vi "mediaIntesecaoCameras_v2.vi"(11 "Cameras Array":T1[](array[typedef]) {"robots_blue"."height" format="%+4.3f"; "robots_blue"."pixel_y" format="%+4.3f"; "robots_blue"."pixel_x" format="%+4.3f"; "robots_blue"."orientation" format="%+4.3f"; "robots_blue"."y" format="%+4.3f"; "robots_blue"."confidence" format="%4.3f"; "robots_blue"."x" format="%+4.3f"; "robots_yellow"."height" format="%+4.3f"; "robots_yellow"."pixel_y" format="%+4.3f"; "robots_yellow"."pixel_x" format="%+4.3f"; "robots_yellow"."orientation" format="%+4.3f"; "robots_yellow"."y" format="%+4.3f"; "robots_yellow"."confidence" format="%4.3f"; "robots_yellow"."x" format="%+4.3f"}) -> (3 "frame out":T1 {"robots_blue"."height" format="%+4.3f"; "robots_blue"."pixel_y" format="%+4.3f"; "robots_blue"."pixel_x" format="%+4.3f"; "robots_blue"."orientation" format="%+4.3f"; "robots_blue"."y" format="%+4.3f"; "robots_blue"."confidence" format="%4.3f"; "robots_blue"."x" format="%+4.3f"; "robots_yellow"."height" format="%+4.3f"; "robots_yellow"."pixel_y" format="%+4.3f"; "robots_yellow"."pixel_x" format="%+4.3f"; "robots_yellow"."orientation" format="%+4.3f"; "robots_yellow"."y" format="%+4.3f"; "robots_yellow"."confidence" format="%4.3f"; "robots_yellow"."x" format="%+4.3f"})   [LabVIEW 2018]
uses:
  SSL Detection Frame.ctl
  SSL Detection Robot.ctl
  <vilib>/Analysis/Matrix/Datatypes/RealMatrix.ctl
  SSL Detection Ball.ctl
  <vilib>/Analysis/Matrix/NI_Matrix.lvlib
panel:
  in  "Unico frame":T1 {"robots_blue"."height" format="%+4.3f"; "robots_blue"."pixel_y" format="%+4.3f"; "robots_blue"."pixel_x" format="%+4.3f"; "robots_blue"."orientation" format="%+4.3f"; "robots_blue"."y" format="%+4.3f"; "robots_blue"."confidence" format="%4.3f"; "robots_blue"."x" format="%+4.3f"; "robots_yellow"."height" format="%+4.3f"; "robots_yellow"."pixel_y" format="%+4.3f"; "robots_yellow"."pixel_x" format="%+4.3f"; "robots_yellow"."orientation" format="%+4.3f"; "robots_yellow"."y" format="%+4.3f"; "robots_yellow"."confidence" format="%4.3f"; "robots_yellow"."x" format="%+4.3f"}
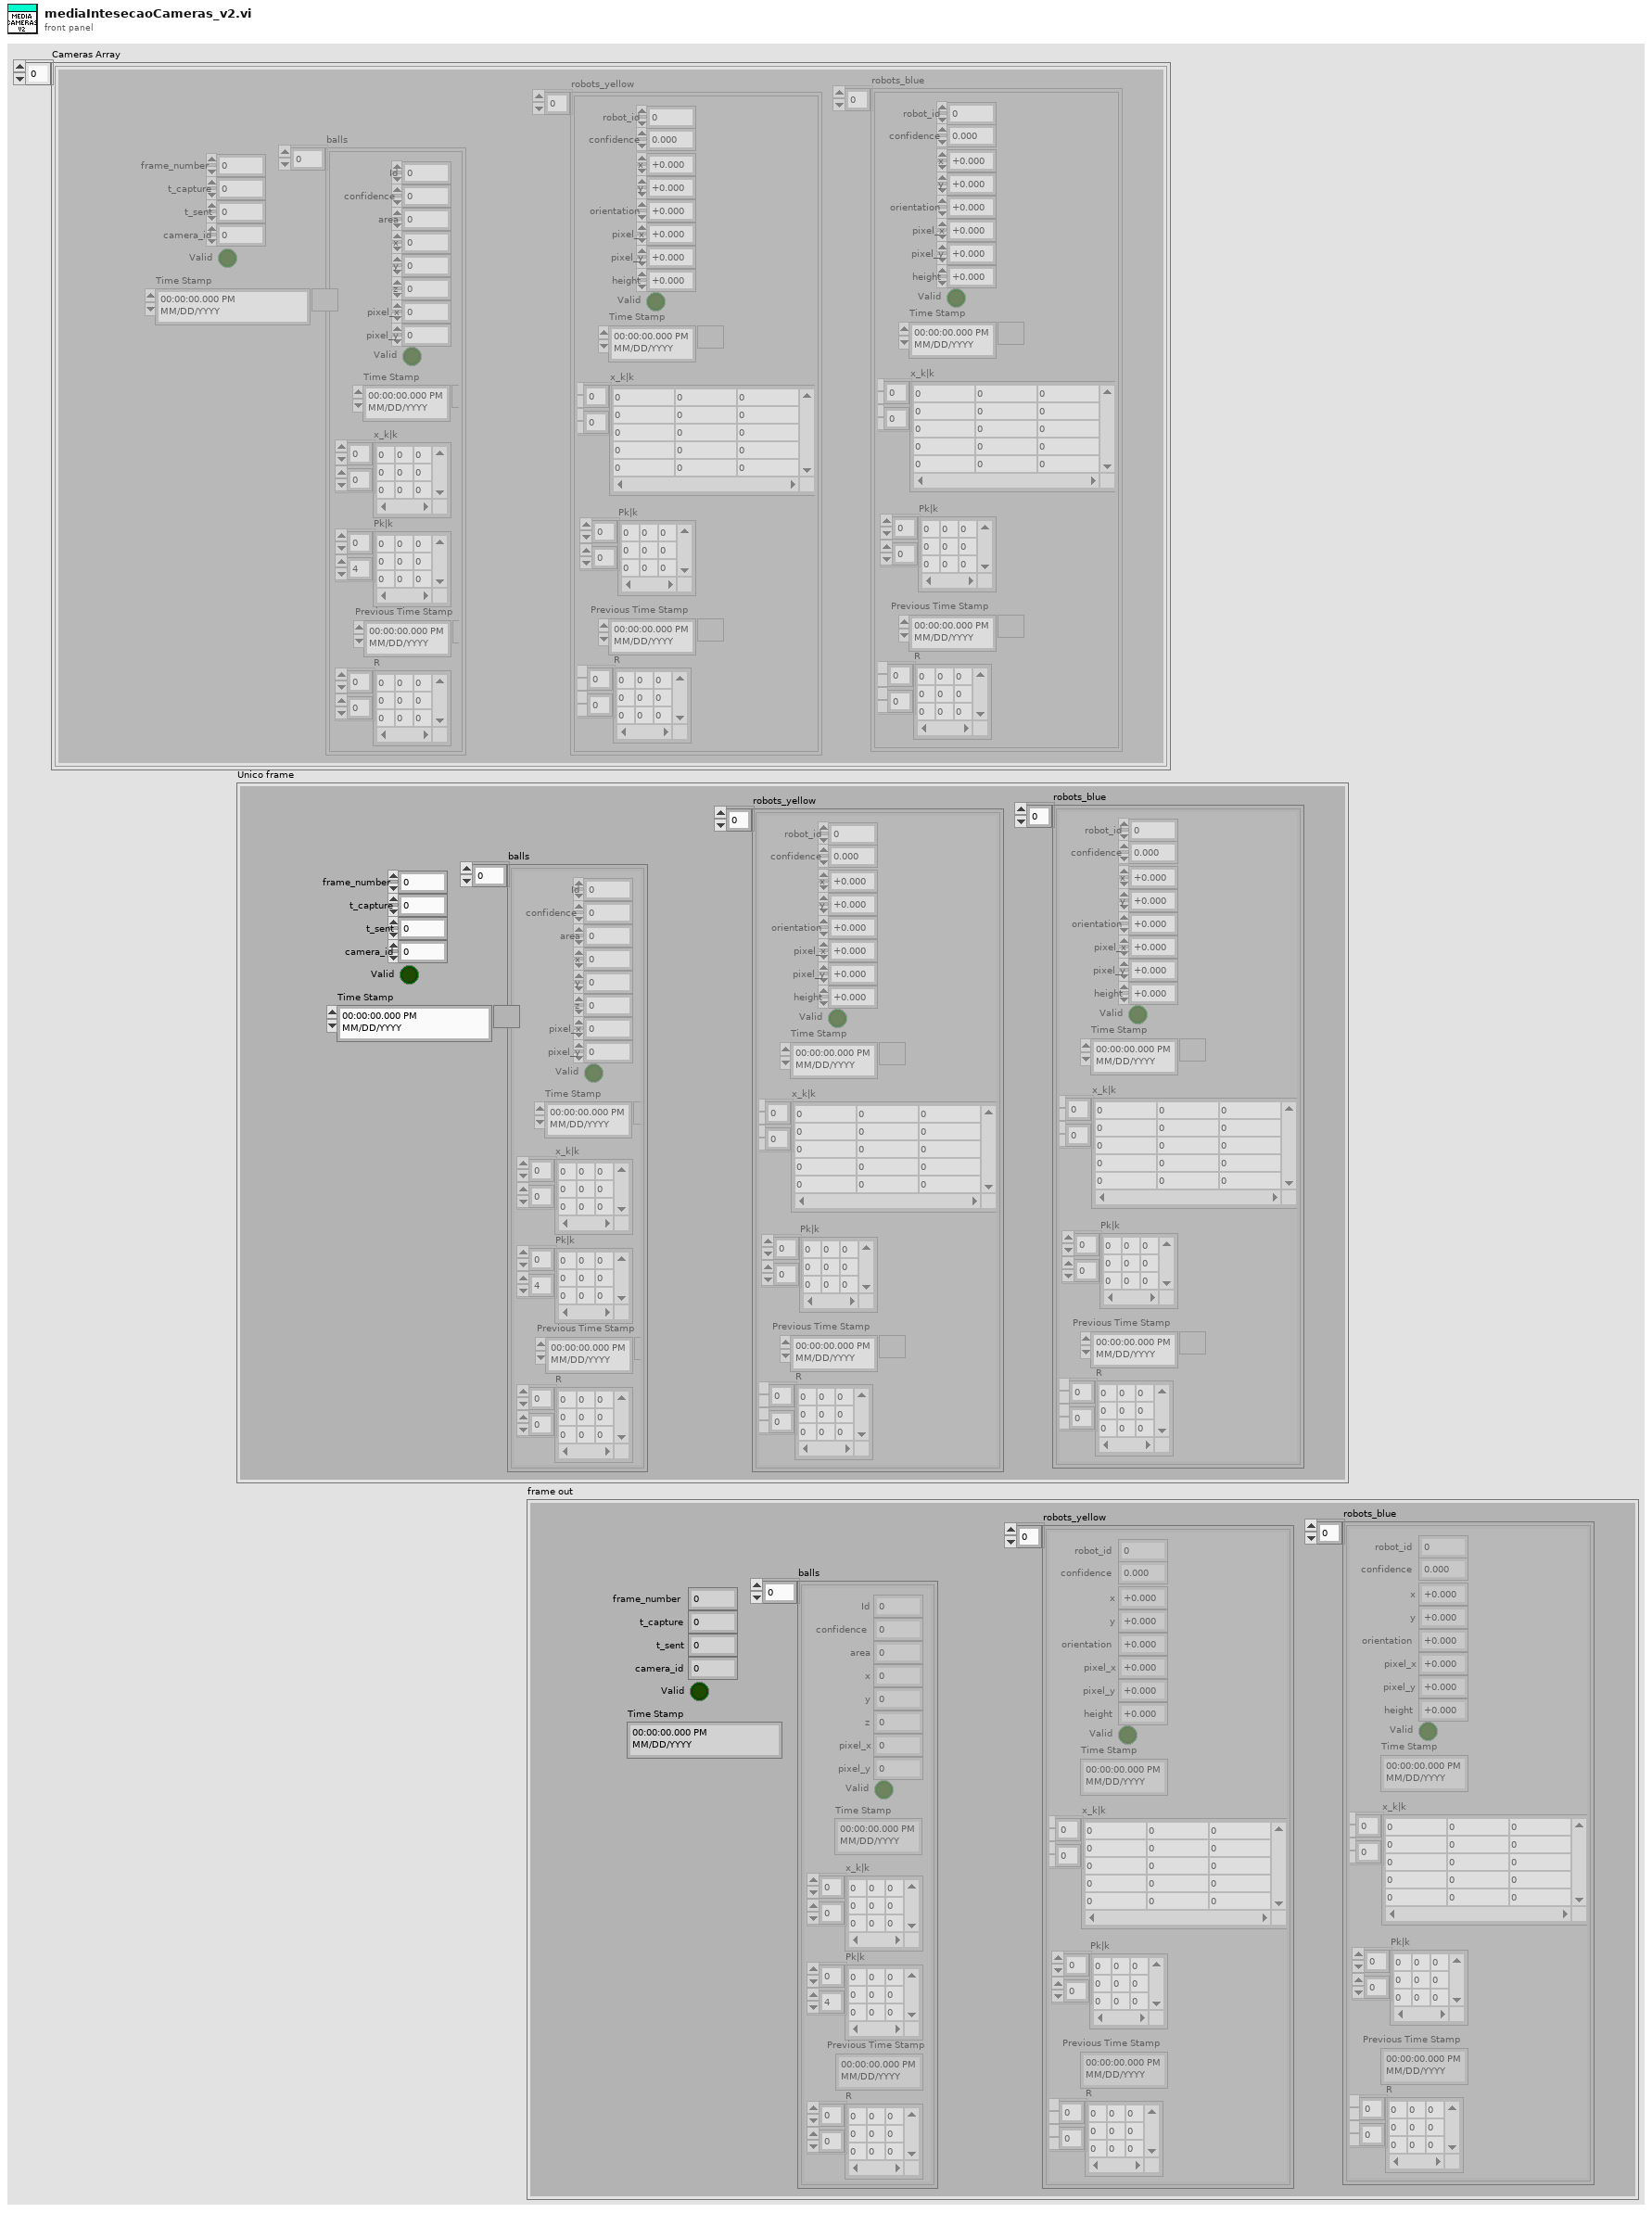
[diagram p1: front panel]
types:
  T1 = typedef "SSL Detection Frame.ctl" = cluster{"frame_number":u32, "t_capture":dbl, "t_sent":dbl, "camera_id":u32, "robots_yellow":T2[], "robots_blue":T2[], "balls":T4[], "Valid":bool, "Time Stamp":timestamp}
  T2 = typedef "SSL Detection Robot.ctl" = cluster{"x":sgl, "robot_id":u32, "confidence":sgl, "y":sgl, "orientation":sgl, "pixel_x":sgl, "pixel_y":sgl, "height":sgl, "Valid":bool, "Time Stamp":timestamp, "x_k|k":T3, "Pk|k":T3, "Previous Time Stamp":timestamp, "R":T3}
  T3 = typedef "NI_Matrix.lvlib/RealMatrix.ctl" = dbl[][]
  T4 = typedef "SSL Detection Ball.ctl" = cluster{"x":sgl, "area":u32, "confidence":sgl, "y":sgl, "z":sgl, "pixel_x":sgl, "pixel_y":sgl, "Valid":bool, "Time Stamp":timestamp, "x_k|k":T3, "Pk|k":T3, "Id":u32, "Previous Time Stamp":timestamp, "R":T3}
  T5 = cluster{"x":sgl, "y":sgl, "orientation":sgl, "robot_id":u32, "camera_id":u32}
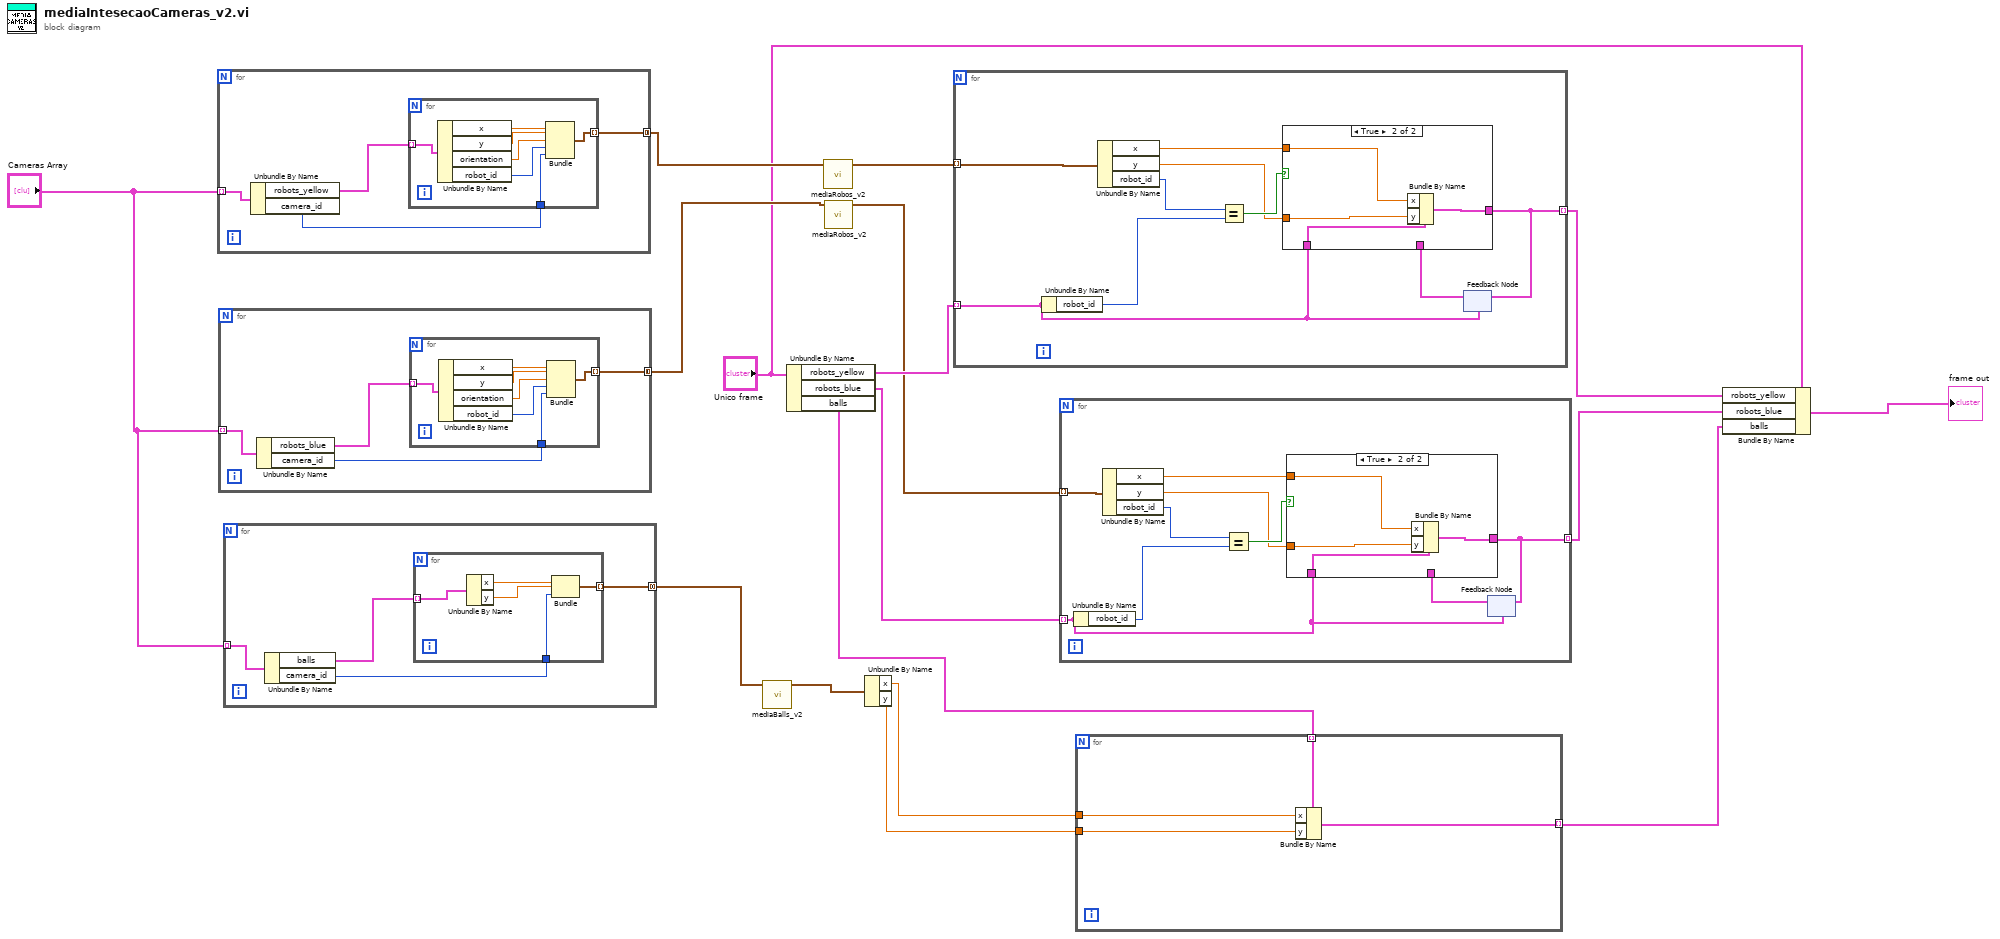
[diagram p0: block diagram]
diagram:
  n1 = for {
    tunnel: "Cameras Array" -> [w21] mode=indexing
    tunnel: [w19] -> w17 mode=concatenating
    n2 = Unbundle By Name(w21) -> ("robots_yellow"=w20:T2[], "camera_id"=w18:u32)
    n3 = for {
      tunnel: w20 -> [w28] mode=indexing
      tunnel: [w25] -> w19 mode=indexing
      tunnel: w18 -> [w22]
      n4 = Unbundle By Name(w28) -> ("x"=w27:sgl, "y"=w26:sgl, "orientation"=w24:sgl, "robot_id"=w23:u32)
      n5 = Bundle("x"=w27, "y"=w26, "orientation"=w24, "robot_id"=w23, "camera_id"=w22) -> (w25:T5)  [unwired: 1 in]
    }
  }
  n6 = for {
    tunnel: "Cameras Array" -> [w32] mode=indexing
    tunnel: [w31] -> w12 mode=concatenating
    n7 = Unbundle By Name(w32) -> ("robots_blue"=w29:T2[], "camera_id"=w30:u32)
    n8 = for {
      tunnel: w29 -> [w39] mode=indexing
      tunnel: [w36] -> w31 mode=indexing
      tunnel: w30 -> [w33]
      n9 = Unbundle By Name(w39) -> ("x"=w38:sgl, "y"=w37:sgl, "orientation"=w35:sgl, "robot_id"=w34:u32)
      n10 = Bundle("x"=w38, "y"=w37, "orientation"=w35, "robot_id"=w34, "camera_id"=w33) -> (w36:T5)  [unwired: 1 in]
    }
  }
  n11 = for {
    tunnel: "Cameras Array" -> [w43] mode=indexing
    tunnel: [w42] -> w6 mode=concatenating
    n12 = Unbundle By Name(w43) -> ("balls"=w40:T4[], "camera_id"=w41:u32)
    n13 = for {
      tunnel: w40 -> [w48] mode=indexing
      tunnel: [w45] -> w42 mode=indexing
      tunnel: w41 -> [w44]
      n14 = Unbundle By Name(w48) -> ("x"=w47:sgl, "y"=w46:sgl)
      n15 = Bundle("x"=w47, "y"=w46, "camera_id"=w44) -> (w45:cluster{"x":sgl, "y":sgl, "camera_id":u32})  [unwired: 1 in]
    }
  }
  n16 = call "mediaBalls_v2.vi"("Array Ball Pose + CamID"=w6) -> ("Ball out"=w5:cluster{"x":dbl, "y":dbl})  [unwired: 10 in]
  n17 = Unbundle By Name("Unico frame") -> ("robots_yellow"=w16:T2[], "robots_blue"=w14:T2[], "balls"=w4:T4[])
  n18 = call "mediaRobos_v2.vi"("Array Robot Pose + CamID"=w17) -> ("Array"=w15:cluster{"x":dbl, "y":dbl, "robot_id":i32}[])  [unwired: 10 in]
  n19 = call "mediaRobos_v2.vi"("Array Robot Pose + CamID"=w12) -> ("Array"=w13:cluster{"x":dbl, "y":dbl, "robot_id":i32}[])  [unwired: 10 in]
  n20 = Unbundle By Name(w5) -> ("x"=w3:dbl, "y"=w2:dbl)
  n21 = for {
    tunnel: w16 -> [w49] mode=indexing
    tunnel: w15 -> [w56] mode=indexing
    tunnel: [w51] -> w10 mode=indexing
    n22 = Unbundle By Name(w49) -> ("robot_id"=w57:u32)
    n23 = Unbundle By Name(w56) -> ("x"=w53:dbl, "y"=w52:dbl, "robot_id"=w55:i32)
    n24 = Equal?(x=w55, y=w57) -> (x = y?=w54:bool)
    n25 = feedback #1(w49) -> (w50:T2)
    n26 = case shown="True" w54 {
      tunnel: w49 -> [_ w62]
      tunnel: w53 -> [_ w61]
      tunnel: w52 -> [_ w60]
      tunnel: [w58 w59] -> w51
      tunnel: w50 -> [w58 _]
      frame False {
      }
      frame True {
        n27 = Bundle By Name(cluster=w62, "x"=w61, "y"=w60) -> (w59:T2)
      }
    }
    n28 = feedback-in #1(w51) -> ()
  }
  n29 = for {
    tunnel: w14 -> [w63] mode=indexing
    tunnel: w13 -> [w70] mode=indexing
    tunnel: [w65] -> w9 mode=indexing
    n30 = Unbundle By Name(w63) -> ("robot_id"=w71:u32)
    n31 = Unbundle By Name(w70) -> ("x"=w67:dbl, "y"=w66:dbl, "robot_id"=w69:i32)
    n32 = Equal?(x=w69, y=w71) -> (x = y?=w68:bool)
    n33 = feedback #2(w63) -> (w64:T2)
    n34 = case shown="True" w68 {
      tunnel: w63 -> [_ w76]
      tunnel: w67 -> [_ w75]
      tunnel: w66 -> [_ w74]
      tunnel: [w72 w73] -> w65
      tunnel: w64 -> [w72 _]
      frame False {
      }
      frame True {
        n35 = Bundle By Name(cluster=w76, "x"=w75, "y"=w74) -> (w73:T2)
      }
    }
    n36 = feedback-in #2(w65) -> ()
  }
  n37 = for {
    tunnel: w4 -> [w80] mode=indexing
    tunnel: w3 -> [w79]
    tunnel: w2 -> [w78]
    tunnel: [w77] -> w1 mode=indexing
    n38 = Bundle By Name(cluster=w80, "x"=w79, "y"=w78) -> (w77:T4)
  }
  n39 = Bundle By Name(cluster="Unico frame", "robots_yellow"=w10, "robots_blue"=w9, "balls"=w1) -> (→"frame out":T1)
